vi "SinglePoint-GetChannelRefs.vi"(8 "Error in":errorcluster, 9 "Enabled?":bool, 11 "Device Ref in":T2 format="%.0x") -> (0 "Error out":errorcluster, 2 "Result Ch Data Refs":T1[](array[typedef]) format="%.0x", 3 "Device Ref out":T2=18446744073709551615 format="%.0x")   [LabVIEW 2014, in "Waveform-Processing-Custom-Device Shared.lvlib" / "SinglePoint.lvlib"]
uses:
  SinglePoint.lvlib
  <vilib>/NI Veristand/Custom Device API/Custom Device Item Ref.ctl
  <vilib>/NI Veristand/Custom Device API/Data Reference.ctl
  <vilib>/NI Veristand/Custom Device API/Data Access Type.ctl
  Constants.vi
  <vilib>/NI Veristand/Custom Device API/Get Item Property (Dependent Node Pointer).vi
  System Explorer/Waveform-Processing-Custom-Device System Explorer.lvlib
  <vilib>/NI Veristand/Custom Device API/Custom Device API.lvlib
  Waveform-Processing-Custom-Device Shared.lvlib
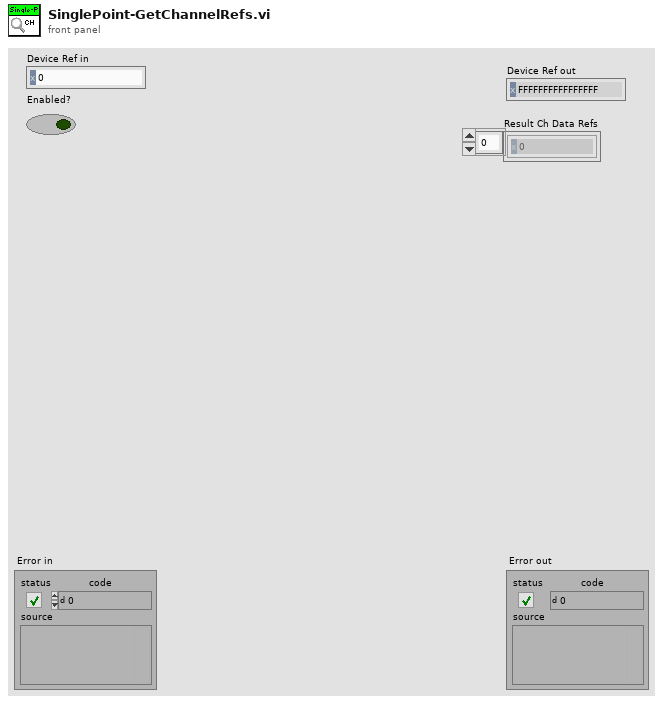
[diagram p1: front panel]
types:
  T1 = typedef "Custom Device API.lvlib/Data Reference.ctl" = i32
  T2 = typedef "Custom Device API.lvlib/Custom Device Item Ref.ctl" = u64
  T3 = typedef "Custom Device API.lvlib/Data Access Type.ctl" = enum16{"Read", "Write"}
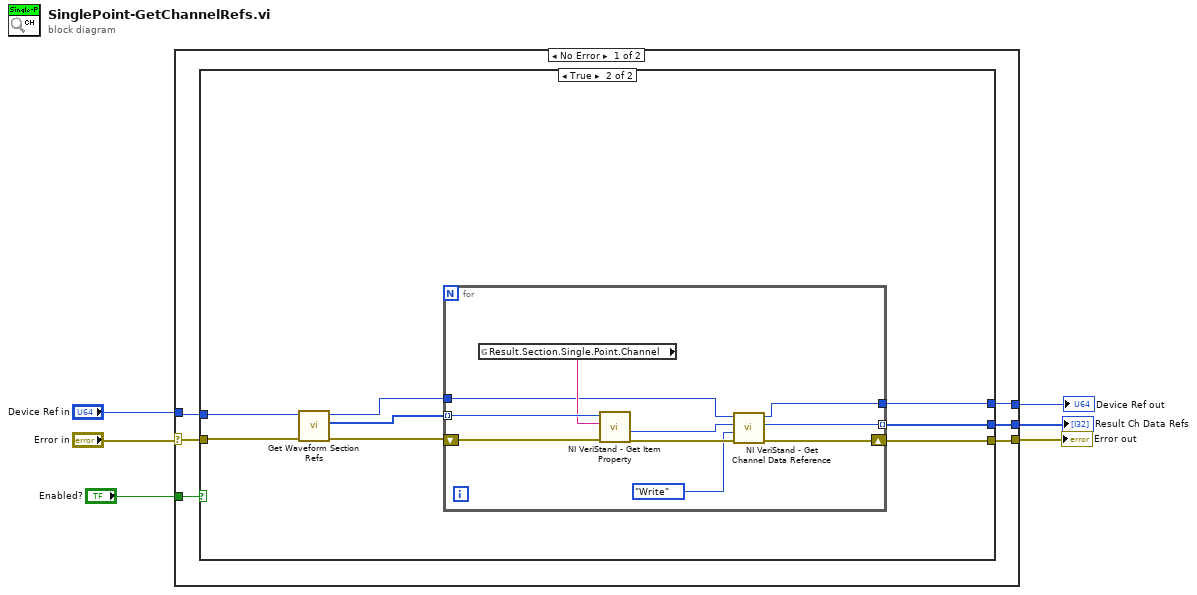
[diagram p0: block diagram]
diagram:
  n1 = case shown="No Error" "Error in" {
    selector: "Error in" -> [w12 w34]
    tunnel: [w10 w34] -> w3
    tunnel: "Device Ref in" -> [w11 w33]
    tunnel: "Enabled?" -> [w9 _]
    tunnel: [w8 w33] -> w6
    tunnel: [w7 _] -> w1
    frame No Error {
      n2 = case shown="True" w9 {
        tunnel: w12 -> [w14 w22]
        tunnel: w11 -> [w13 w21]
        tunnel: [w14 w17] -> w10
        tunnel: [w13 w15] -> w8
        tunnel: [_ w16] -> w7
        frame False {
        }
        frame True {
          n3 = call "Get Waveform Section Refs.vi"("Error in"=w22, "Device Ref in"=w21) -> ("Error out"=w20:errorcluster, "Result Section Refs"=w19:T2[], "Device Ref out"=w18:T2)  [unwired: 7 in]
          n4 = for {
            tunnel: w19 -> [w31] mode=indexing
            tunnel: w18 -> [w27]
            shift-right: [w26] -> w17
            shift-left: w20 -> [w32]
            tunnel: [w25] -> w16 mode=indexing
            tunnel: [w24] -> w15
            n5 = global read "Constants.vi" "Result.Section.Single.Point.Channel"() -> (w30:string)
            n6 = call-poly <vilib>:"NI VeriStand - Get Item Property.vi"("error in (no error)"=w32, "Property Name"=w30, "Item Ref in"=w31) -> ("error out"=w29:errorcluster, "Dependent Node Ref"=w28:T2)  [unwired: 5 in, 2 out]
            n7 = call <vilib>:"NI VeriStand - Get Channel Data Reference.vi"("error in (no error)"=w29, "Access"=Data_Access_Type."Write", "Channel Ref in"=w28, "Device Ref in"=w27) -> ("error out"=w26:errorcluster, "Channel Data Reference"=w25:T1, "Device Ref out"=w24:T2)  [unwired: 5 in]
          }
        }
      }
    }
    frame Error {
    }
  }
  "Error out" <- w3
  "Device Ref out" <- w6
  "Result Ch Data Refs" <- w1
